vi "Export All Mappings.vi"(8 "error in (no error)":errorcluster, 10 "Path":path, 11 "SDF Ref":refnum<k24>) -> (0 "error out":errorcluster)   [LabVIEW 2016, in "System Mapping Tool.lvlib"]
uses:
  System Mapping Tool.lvlib
  NationalInstruments.VeriStand.SystemDefinitionAPI
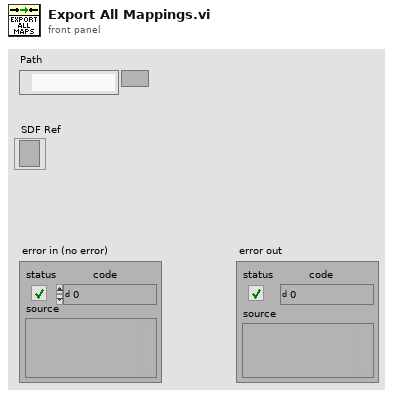
[diagram p1: front panel]
types:
  T1 = enum16{"open", "replace", "create", "open or create", "replace or create", "replace or create with confirmation"}
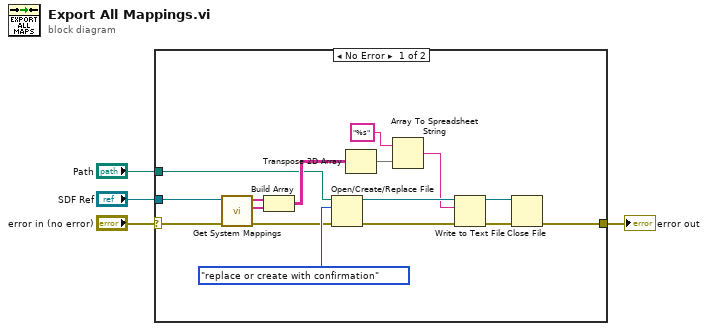
[diagram p0: block diagram]
diagram:
  n1 = case shown="No Error" "error in (no error)" {
    selector: "error in (no error)" -> [w10 w21]
    tunnel: [w6 w21] -> w3
    tunnel: "SDF Ref" -> [w9 _]
    tunnel: "Path" -> [w5 _]
    frame No Error {
      n2 = call "Get System Mappings.vi"("error in (no error)"=w10, "SDF Ref"=w9) -> ("error out"=w8:errorcluster, "Destinations"=w18:string[], "Sources"=w19:string[])  [unwired: 7 in]
      n3 = Build Array(w19, w18) -> (w17:string[][])
      n4 = Open/Create/Replace File(file path (use dialog)=w5, error in=w8, operation (0:open)=T1."replace or create with confirmation") -> (refnum out=w15:refnum<file>, error out=w7:errorcluster)  [unwired: 3 in, 1 out]
      n5 = Transpose 2D Array(2D array=w17) -> (transposed array=w11:string[][])
      n6 = Array To Spreadsheet String(array=w11, 3:"%s" ("format string")) -> (spreadsheet string=w14:string)  [unwired: 1 in]
      n7 = Write to Text File(file (use dialog)=w15, text=w14, error in=w7) -> (refnum out=w12:refnum<file>, error out=w13:errorcluster)  [unwired: 1 in, 1 out]
      n8 = Close File(refnum=w12, error in=w13) -> (error out=w6:errorcluster)  [unwired: 1 out]
    }
    frame Error {
    }
  }
  "error out" <- w3
